vi "PV Software LDO Trigger Temperature.vi"(11 "HEX Data (U8)":u8 format="%x") -> (3 "LDO Trigger Temperature":string)   [LabVIEW 2023]
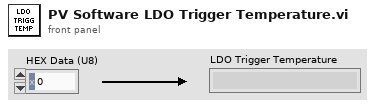
[diagram p1: front panel]
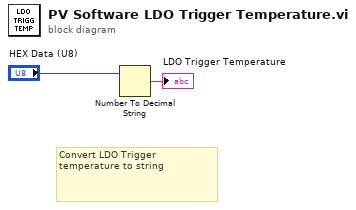
[diagram p0: block diagram]
diagram:
  # "Convert LDO Trigger temperature to string"
  n1 = Number To Decimal String(number="HEX Data (U8)") -> (decimal integer string=→"LDO Trigger Temperature":string)  [unwired: 1 in]
